vi "DSF.Engine.Plugin.Set Thread ID Pool.vi"(10 "Thread ID Pool":refnum<class "DSF.Engine.Pool.ID.lvclass">, 11 "Plugin in":refnum<class "Plugin.lvclass">) -> (3 "Plugin out":refnum<class "Plugin.lvclass">)   [LabVIEW 2017, in "DSF.Engine.lvlib" / "Plugin.lvclass"]
uses:
  Plugin.lvclass
  Thread Pool/DSF.Engine.Pool.ID.lvclass
  Plugin.lvclass/Plugin.ctl
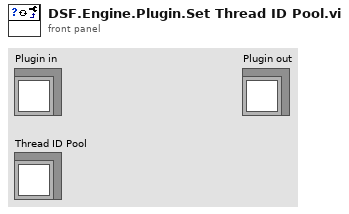
[diagram p1: front panel]
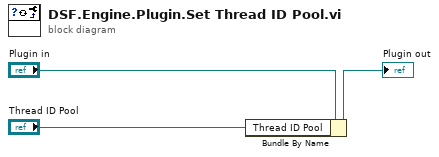
[diagram p0: block diagram]
diagram:
  n1 = Bundle By Name(cluster="Plugin in", "Thread ID Pool"="Thread ID Pool") -> (→"Plugin out":refnum<class "Plugin.lvclass">)
